vi "串口-单次读写.vi"(5 "轮询间隔（10ms）":u32=10, 6 "等待字节数(4096)":u32=4096, 7 "确定次数（1）":u32=1, 8 "错误输入（无错误）":errorcluster, 9 "设置超时(默认-1,单位ms)":i32=-1, 10 "写入缓冲区":string, 11 "VISA资源名称":refnum<visa-resource-name>) -> (0 "错误输出":errorcluster, 2 "读取缓冲区":string, 3 "VISA资源名称输出":refnum<visa-resource-name>)   [LabVIEW 2017]
doc: "不包括开关串口, 读写前会清空缓冲区一次."
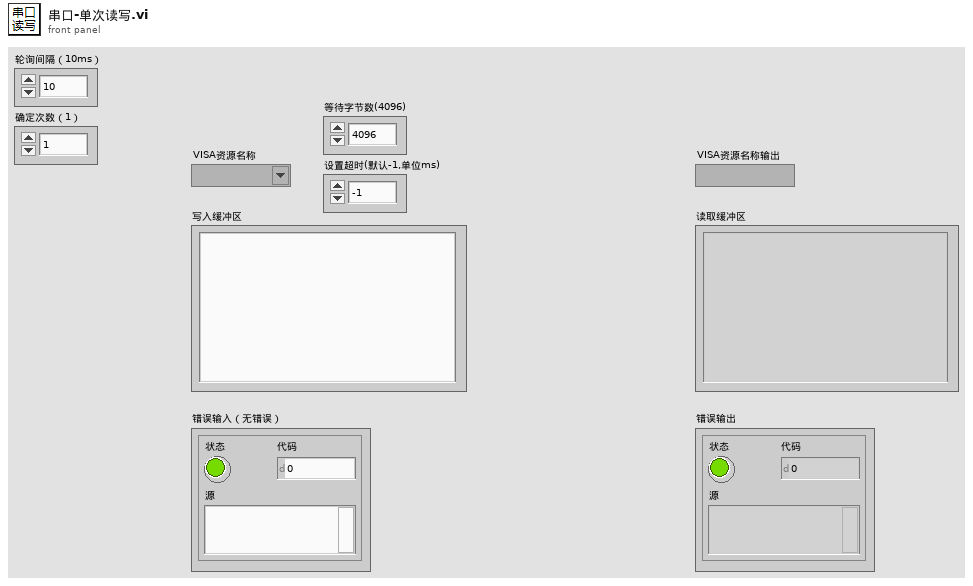
[diagram p1: front panel]
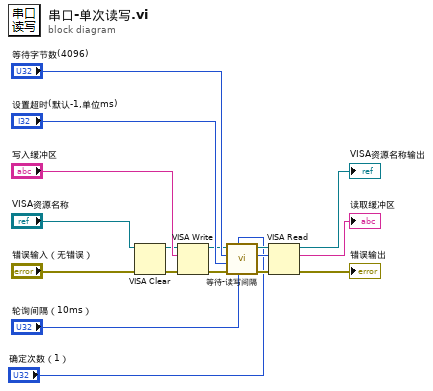
[diagram p0: block diagram]
diagram:
  n1 = VISA Clear(VISA resource name="VISA资源名称", error in (no error)="错误输入（无错误）") -> (VISA resource name out=w7:refnum<visa-resource-name>, error out=w5:errorcluster)
  n2 = VISA Write(VISA resource name=w7, write buffer="写入缓冲区", error in (no error)=w5) -> (VISA resource name out=w9:refnum<visa-resource-name>, error out=w8:errorcluster)  [unwired: 1 out]
  n3 = call "等待-读写间隔.vi"("轮询间隔（10ms）"="轮询间隔（10ms）", "确定次数（1）"="确定次数（1）", "error in"=w8, "设置超时(默认-1,单位ms)"="设置超时(默认-1,单位ms)", "等待字节数(4096)"="等待字节数(4096)", "VISA资源名i"=w9) -> ("error out"=w15:errorcluster, "读取字节数"=w16:u32, "VISA资源名o"=w17:refnum<visa-resource-name>)  [unwired: 1 in, 2 out]
  n4 = VISA Read(VISA resource name=w17, byte count=w16, error in (no error)=w15) -> (VISA resource name out=→"VISA资源名称输出":refnum<visa-resource-name>, read buffer=→"读取缓冲区":string, error out=→"错误输出":errorcluster)  [unwired: 1 out]
